vi "Stack ID in Stack.vi"(8 "error in (no error)":errorcluster, 10 "Stack ID":u8, 11 "Stack in":refnum<class "Device.lvclass">[](array[class])) -> (0 "error out":errorcluster, 1 "Stack Index":i32, 2 "Device found?":bool, 3 "Stack out":refnum<class "Device.lvclass">[](array[class]), 4 "Device out":refnum<class "Device.lvclass">)   [LabVIEW 2011, in "Tinkerforge.lvlib" / "Device.lvclass"]
doc: "This VI searches if the given Stack ID is present in the stack."
uses:
  Device.lvclass
  Device.lvclass/Device.ctl
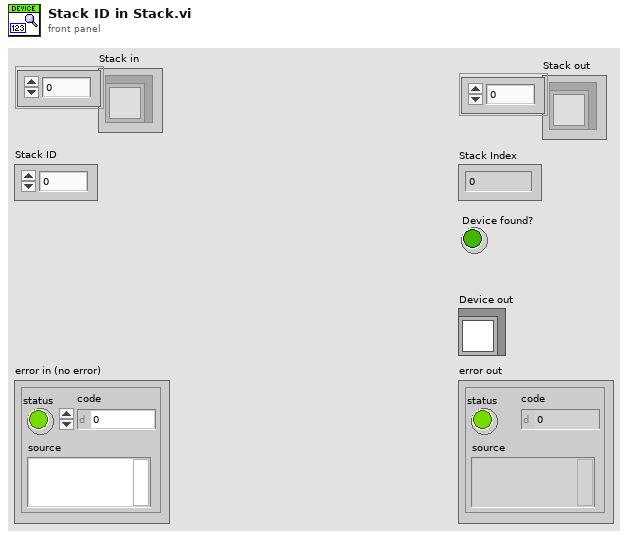
[diagram p1: front panel]
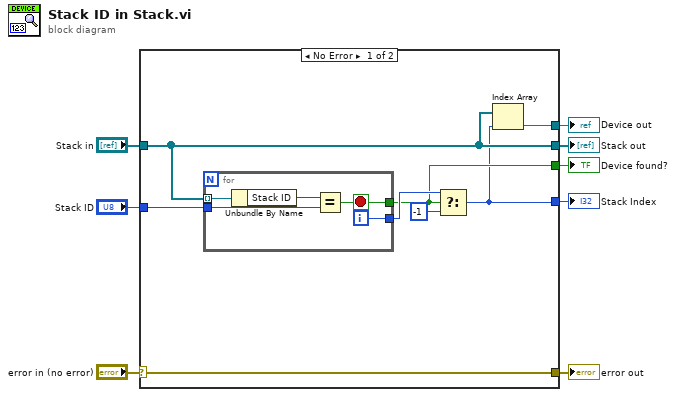
[diagram p0: block diagram]
diagram:
  n1 = case shown="No Error" "error in (no error)" {
    selector: "error in (no error)" -> [w16 w23]
    tunnel: [w16 w23] -> w7
    tunnel: "Stack in" -> [w11 w22]
    tunnel: [w11 w22] -> w5
    tunnel: "Stack ID" -> [w15 _]
    tunnel: [w12 _] -> w3
    tunnel: [w10 _] -> w2
    tunnel: [w9 _] -> w1
    frame No Error {
      n2 = for {
        tunnel: w11 -> [w21] mode=indexing
        tunnel: w15 -> [w19]
        tunnel: [w18] -> w14
        tunnel: [w17] -> w12
        i -> [w18]
        stop <- w17 stop-if-true
        n3 = Unbundle By Name(w21) -> ("Stack ID"=w20:u8)
        n4 = Equal?(x=w20, y=w19) -> (x = y?=w17:bool)
      }
      n5 = Select(t=w14, s=w12, f=-1) -> (s? t:f=w10:i32)
      n6 = Index Array(array=w11, index=w10) -> (element=w9:refnum<class "Device.lvclass">)
    }
    frame Error {
    }
  }
  "error out" <- w7
  "Stack out" <- w5
  "Device found?" <- w3
  "Stack Index" <- w2
  "Device out" <- w1
